vi "Configuration.vi"(6 "Return Data":refnum<user-event>, 8 "error in (no error)":errorcluster, 9 "Exit Running Config":refnum<user-event>, 10 "Panel in":refnum<class "Panel.lvclass">, 11 "Generic Data Type in":refnum<class "Generic Data Type.lvclass">) -> (0 "error out":errorcluster, 3 "Generic Data Type out":refnum<class "Generic Data Type.lvclass">)   [LabVIEW 2018, in "Generic Data Type.lvclass"]
uses:
  Generic Data Type.lvclass
  <vilib>/MGI/Panel Manager/Panel/Panel/Panel.lvclass
panel:
  # "UI for Configuration Goes Here"
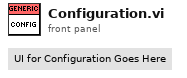
[diagram p1: front panel]
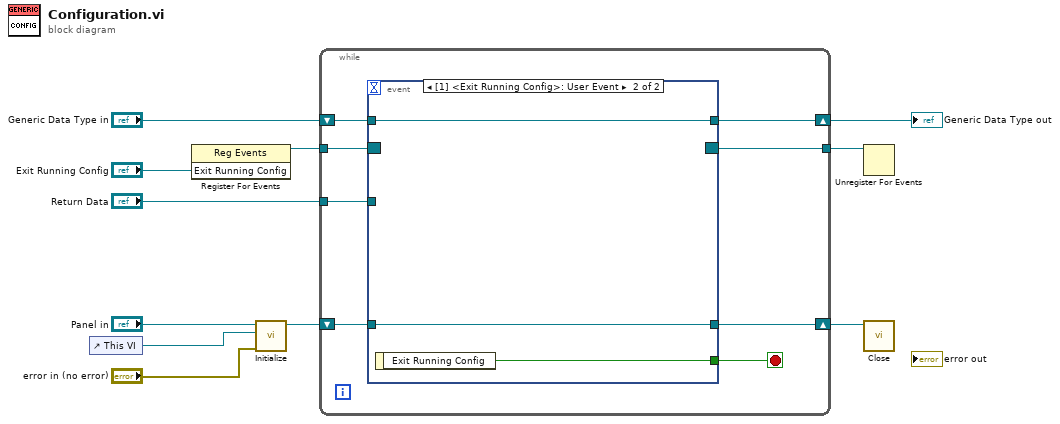
[diagram p0: block diagram]
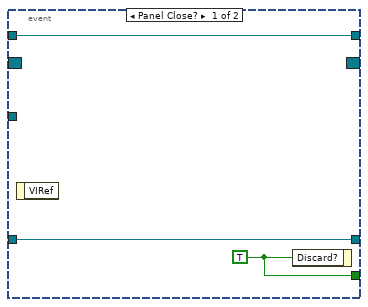
[diagram p2: hidden frame]
diagram:
  n1 = control-ref of="This VI"() -> (w10:refnum<vi>)
  n2 = register-events("Exit Running Config") -> (reference out=w3:refnum<event-registration>)  [unwired: 2 in, 1 out]
  n3 = call <vilib>:"Initialize.vi"("error in (no error)"="error in (no error)", "VI Refnum"=w10, "Panel In"="Panel in") -> ("Panel Out"=w5:refnum<class "Panel.lvclass">)  [unwired: 6 in, 2 out]
  n4 = while {
    shift-right: [w13] -> w6
    shift-left: "Generic Data Type in" -> [w19]
    shift-right: [w15] -> w4
    shift-left: w5 -> [w16]
    tunnel: w3 -> [w17]
    tunnel: [w14] -> w2
    tunnel: "Return Data" -> [w12]
    stop <- w18 stop-if-true
    n5 = event shown="[1] <Exit Running Config>: User Event" {
      selector: w17 -> [_ _]
      dyn-events: [_ _] -> w14
      timeout: _ -> [_ _]
      tunnel: w19 -> [w22 w25]
      tunnel: [w22 w25] -> w13
      tunnel: [w21 w23] -> w18
      tunnel: w16 -> [w20 w24]
      tunnel: [w20 w24] -> w15
      tunnel: w12 -> [_ _]
      event Panel Close? {
        w21 = TRUE
        n6 = event-data() -> ()  [unwired: 1 in, 1 out]
        n7 = event-data("Discard?"=w21) -> ()  [unwired: 1 in, 1 out]
      }
      event User Event {
        n8 = event-data() -> ("Exit Running Config"=w23:bool)  [unwired: 1 in]
      }
    }
  }
  "Generic Data Type out" <- w6
  n9 = Unregister For Events(event registration refnum=w2) -> ()  [unwired: 1 in, 1 out]
  n10 = call-dynamic "Close.vi"("Panel In"=w4) -> ()  [unwired: 10 in, 1 out]
